vi "Stop Core.vi"(10 "final error code":i32, 11 "UserInterface in":refnum<class "UserInterface.lvclass">) -> (3 "UserInterface out":refnum<class "UserInterface.lvclass">)   [LabVIEW 2016, in "UserInterface.lvlib" / "UserInterface.lvclass"]
doc: "(<B>Filename</B>: Actor Framework.lvlib:Actor.lvclass:Stop Core.vi)\n\nDefines what the actor does before it stops. Use the <B>final error code</B> input to determine whether the actor shut down in response to an error.\n\nBy default, this method does nothing. A descendant class may override it to define behavior, such as shutting down any processes the actor initiated in its override of the Actor Core method."
uses:
  UserInterface.lvclass
  UserInterface.lvclass/UserInterface.ctl
  <vilib>/ActorFramework/Actor/Actor.lvclass
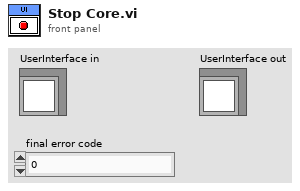
[diagram p1: front panel]
types:
  T1 = enum32{"Invalid", "Standard", "Closed", "Hidden", "Minimized", "Maximized"}
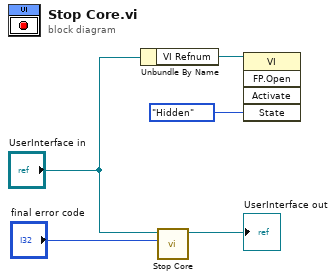
[diagram p0: block diagram]
diagram:
  n1 = Unbundle By Name("UserInterface in") -> ("VI Refnum"=w2:refnum<vi>)
  n2 = call-parent "Stop Core.vi"("final error code"="final error code", "Actor in"="UserInterface in") -> ("Actor out"=→"UserInterface out":refnum<class "UserInterface.lvclass">)  [unwired: 9 in]
  n3 = invoke class="VI" method="FP.Open"(reference=w2, "State"=T1."Hidden") -> ()  [unwired: 3 in, 5 out]
